vi "rgb to grayscale.vi"(7 "Convert Depth?":bool, 8 "error in (no error)":errorcluster, 10 "Processing Params":T1, 11 "Image In":T2) -> (0 "error out":errorcluster, 2 "Depth Values":dbl[][](array[numeric]), 3 "Image Out":T2, 4 "Elapsed Time (ms)":u32)   [LabVIEW 2018]
uses:
  <vilib>/vision/Image Controls.llb/IMAQ Image.ctl
  Processing Params STYP.ctl
  Pixel Data STYP.ctl
  Coordinate STYP.ctl
  Floating Pixel Data STYP.ctl
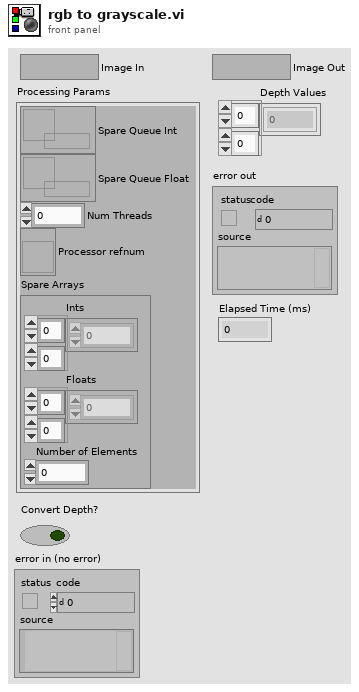
[diagram p1: front panel]
types:
  T1 = typedef "Processing Params STYP.ctl" = cluster{"Spare Queue Int":refnum<queue>, "Spare Queue Float":refnum<queue>, "Num Threads":i32, "Processor refnum":refnum<vi>, "Spare Arrays":cluster{"Ints":u8[][], "Floats":dbl[][], "Number of Elements":i32}}
  T2 = typedef "IMAQ Image.ctl" = refnum<image>
  T3 = typedef "Image Type" = u32
  T4 = typedef "Coordinate STYP.ctl" = cluster{"X":i32, "Y":i32}
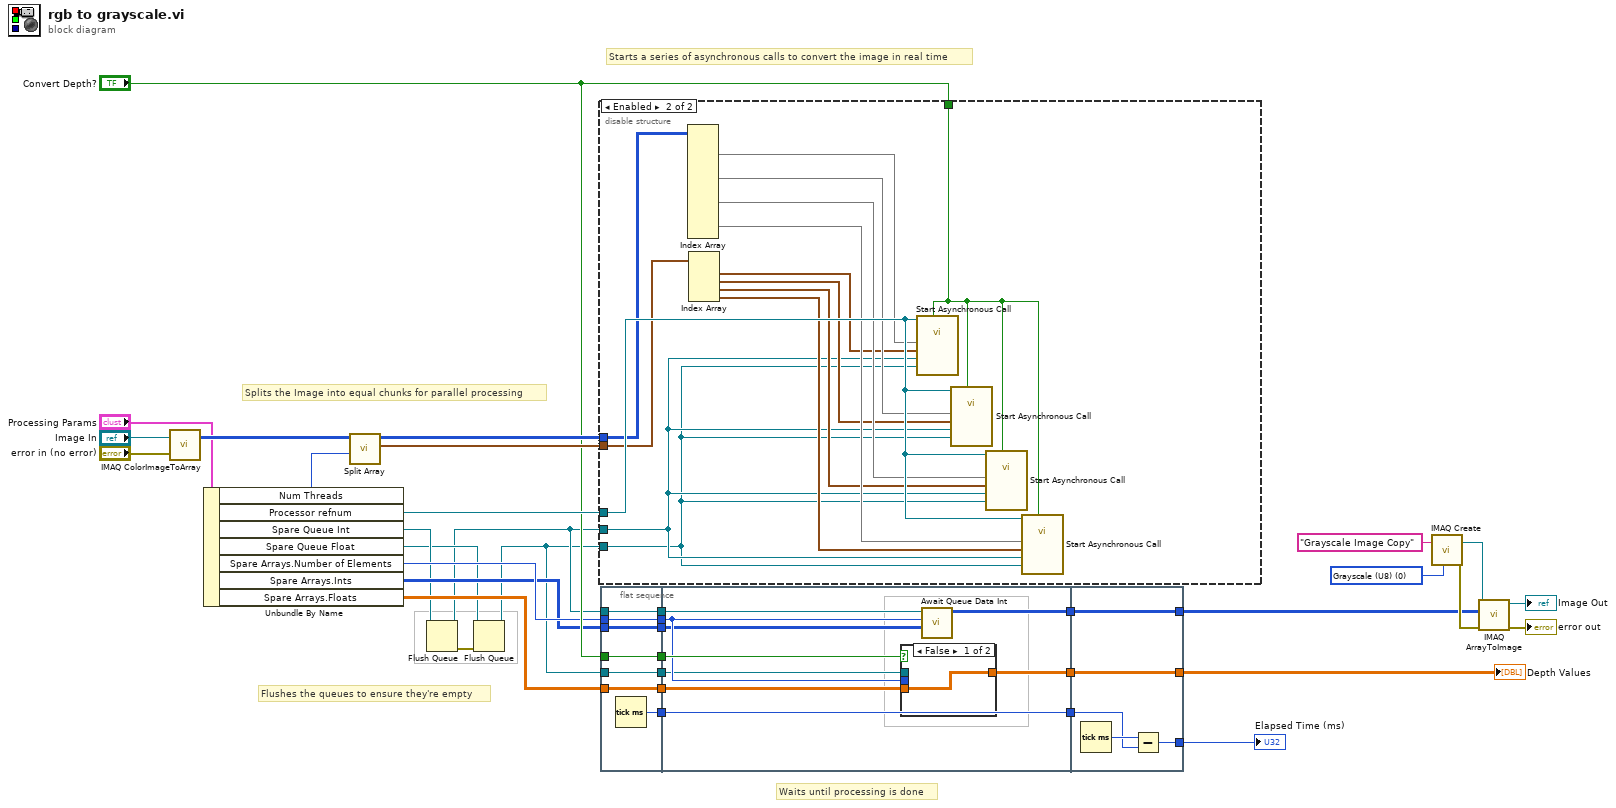
[diagram p0: block diagram]
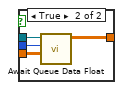
[diagram p2: hidden frame]
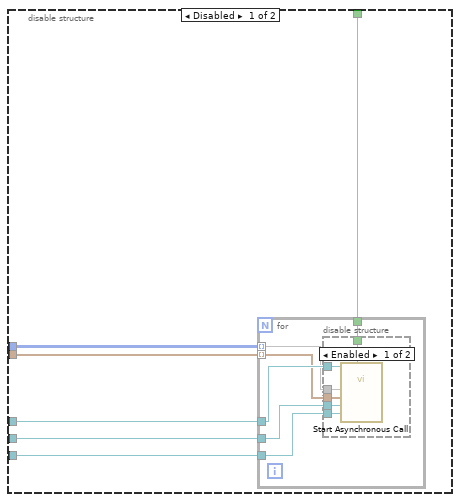
[diagram p3: hidden frame]
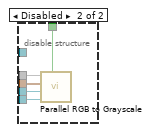
[diagram p4: hidden frame]
diagram:
  w33 = T3 0 items=["Grayscale (U8)", "Grayscale (I16)", "Grayscale (SGL)", "Complex (CSG)", "RGB (U32)", "HSL (U32)", "RGB (U64)", "Grayscale (U16)"] ("Image Type")
  # "Flushes the queues to ensure they're empty"
  # "Splits the Image into equal chunks for parallel processing"
  # "Starts a series of asynchronous calls to convert the image in real time"
  # "Waits until processing is done"
  n1 = call "IMAQ ColorImageToArray"("Image"="Image In", "error in (no error)"="error in (no error)") -> ("Image Pixels (U32)"=w28:u32[][])  [unwired: 2 in, 2 out]
  n2 = Unbundle By Name("Processing Params") -> ("Num Threads"=w26:i32, "Processor refnum"=w23:refnum<vi>, "Spare Queue Int"=w17:refnum<queue>, "Spare Queue Float"=w16:refnum<queue>, "Spare Arrays.Number of Elements"=w21:i32, "Spare Arrays.Ints"=w20:u8[][], "Spare Arrays.Floats"=w19:dbl[][])
  n3 = call "Split Array.vi"("Number of Segments"=w26, "Array"=w28) -> ("Offsets"=w24:T4[], "Split Array"=w25:u32[][][])  [unwired: 8 in]
  n4 = Flush Queue(queue=w17) -> (queue out=w15:refnum<queue>, error out=w12:errorcluster)  [unwired: 1 in, 1 out]
  n5 = Flush Queue(queue=w16, error in (no error)=w12) -> (queue out=w14:refnum<queue>)  [unwired: 2 out]
  n6 = disable-structure shown="Enabled" {
    disable-tunnel: w25 -> [w42 w71]
    disable-tunnel: w24 -> [w41 w70]
    disable-tunnel: w23 -> [w40 w72]
    disable-tunnel: "Convert Depth?" -> [w39 w73]
    disable-tunnel: w15 -> [w38 w61]
    disable-tunnel: w14 -> [w37 w60]
    frame Disabled {
      n7 = for {
        tunnel: w42 -> [w47] mode=indexing
        tunnel: w41 -> [w46] mode=indexing
        tunnel: w40 -> [w48]
        tunnel: w38 -> [w45]
        tunnel: w37 -> [w44]
        tunnel: w39 -> [w43]
        n8 = disable-structure shown="Enabled" {
          disable-tunnel: w48 -> [w54 _]
          disable-tunnel: w47 -> [w53 w59]
          disable-tunnel: w46 -> [w52 w57]
          disable-tunnel: w45 -> [w51 w56]
          disable-tunnel: w44 -> [w50 w55]
          disable-tunnel: w43 -> [w49 w58]
          frame Enabled {
            n9 = call-by-ref "Start Asynchronous Call"(reference=w54, "Depth?"=w49, "Pixel Queue Float"=w50, "Pixel Queue"=w51, "Coordinate"=w52, "Image Pixels (U32)"=w53) -> ()  [unwired: 8 in, 2 out]
          }
          frame Disabled {
            n10 = call "Parallel RGB to Grayscale.vi"("Depth?"=w58, "Pixel Queue Float"=w55, "Pixel Queue"=w56, "Coordinate"=w57, "Image Pixels (U32)"=w59) -> ()  [unwired: 7 in]
          }
        }
      }
    }
    frame Enabled {
      n11 = Index Array(array=w71) -> (element #1=w69:u32[][], element #2=w68:u32[][], element #3=w67:u32[][], element #4=w66:u32[][])  [unwired: 12 in]
      n12 = Index Array(array=w70) -> (element #1=w65:T4, element #2=w64:T4, element #3=w63:T4, element #4=w62:T4)  [unwired: 4 in]
      n13 = call-by-ref "Start Asynchronous Call"(reference=w72, "Depth?"=w73, "Pixel Queue Float"=w60, "Pixel Queue"=w61, "Coordinate"=w65, "Image Pixels (U32)"=w69) -> ()  [unwired: 8 in, 2 out]
      n14 = call-by-ref "Start Asynchronous Call"(reference=w72, "Depth?"=w73, "Pixel Queue Float"=w60, "Pixel Queue"=w61, "Coordinate"=w64, "Image Pixels (U32)"=w68) -> ()  [unwired: 8 in, 2 out]
      n15 = call-by-ref "Start Asynchronous Call"(reference=w72, "Depth?"=w73, "Pixel Queue Float"=w60, "Pixel Queue"=w61, "Coordinate"=w63, "Image Pixels (U32)"=w67) -> ()  [unwired: 8 in, 2 out]
      n16 = call-by-ref "Start Asynchronous Call"(reference=w72, "Depth?"=w73, "Pixel Queue Float"=w60, "Pixel Queue"=w61, "Coordinate"=w62, "Image Pixels (U32)"=w66) -> ()  [unwired: 8 in, 2 out]
    }
  }
  n17 = flat-sequence {
    tunnel: w14 -> [w75]
    tunnel: w15 -> [w76]
    tunnel: w19 -> [w77]
    tunnel: w20 -> [w78]
    tunnel: w21 -> [w79]
    tunnel: "Convert Depth?" -> [w80]
    tunnel: [w80] -> w11
    tunnel: [w79] -> w10
    tunnel: [w78] -> w9
    tunnel: [w77] -> w8
    tunnel: [w76] -> w7
    tunnel: [w75] -> w6
    tunnel: [w74] -> w3
    tunnel: w11 -> [w89]
    tunnel: w10 -> [w88]
    tunnel: w9 -> [w87]
    tunnel: w8 -> [w86]
    tunnel: w7 -> [w84]
    tunnel: w6 -> [w83]
    tunnel: [w85] -> w5
    tunnel: [w82] -> w4
    tunnel: w3 -> [w81]
    tunnel: [w81] -> w2
    tunnel: [w98] -> w13
    tunnel: [w99] -> w18
    tunnel: w5 -> [w99]
    tunnel: w4 -> [w98]
    tunnel: w2 -> [w96]
    tunnel: [w95] -> w1
    frame #0 {
      n18 = Tick Count (ms)() -> (millisecond timer value=w74:u32)
    }
    frame #1 {
      n19 = case shown="False" w89 {
        tunnel: w83 -> [_ w94]
        tunnel: w88 -> [_ w93]
        tunnel: w86 -> [w90 w92]
        tunnel: [w90 w91] -> w82
        frame False {
        }
        frame True {
          n20 = call "Await Queue Data Float.vi"("Array"=w92, "Num Elements"=w93, "Spare Queue Float"=w94) -> ("Array Out"=w91:dbl[][])  [unwired: 8 in]
        }
      }
      n21 = call "Await Queue Data Int.vi"("Array"=w87, "Num Elements"=w88, "Spare Queue Int"=w84) -> ("Array Out"=w85:u8[][])  [unwired: 8 in]
    }
    frame #2 {
      n22 = Tick Count (ms)() -> (millisecond timer value=w97:u32)
      n23 = Subtract(x=w97, y=w96) -> (x-y=w95:u32)
    }
  }
  n24 = call "IMAQ Create"("Image Name"="Grayscale Image Copy", "Image Type"=w33) -> ("New Image"=w32:T2, "error out"=w31:errorcluster)  [unwired: 3 in]
  n25 = call "IMAQ ArrayToImage"("error in (no error)"=w31, "Image Pixels (U8)"=w18, "Image"=w32) -> ("error out"=→"error out":errorcluster, "Image Out"=→"Image Out":T2)  [unwired: 7 in]
  "Depth Values" <- w13
  "Elapsed Time (ms)" <- w1
